vi "Set Message Methods icon without Maker.vi"() -> ()   [LabVIEW 2020]
uses:
  <vilib>/picture/picture.llb/imagedata.ctl
  <vilib>/Utility/traverseref.llb/TRef TravTarget.ctl
  <vilib>/Utility/traverseref.llb/VI Scripting - Traverse.lvlib
panel:
  in  "My Computer?":bool
  in  "Project Path":path
  out "Icon List":picture[](array[picture])
  out "Error List":string[](array[string])
  in  "Folder Path":path
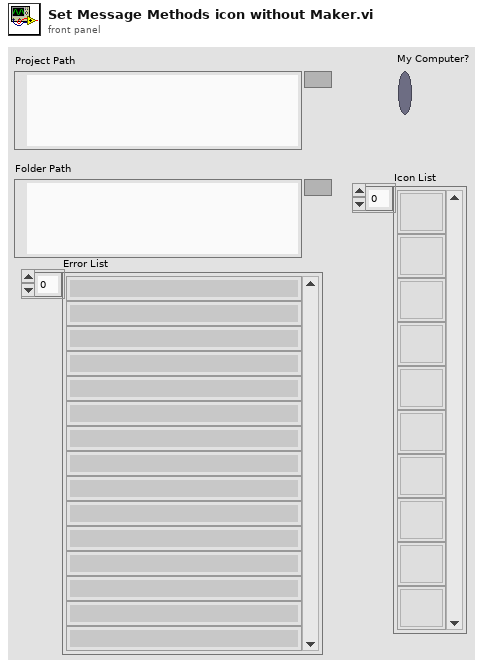
[diagram p1: front panel]
types:
  T1 = enum16{"Set Library Icon", "Get Do Core VI Icon", "Set Private Data Icon", "Set Send VI IIcon"}
  T2 = typedef "imagedata.ctl" = cluster{"image type":i32, "image depth":i32, "image":u8[], "mask":u8[], "colors":u32[], "Rectangle":cluster{"left":i16, "top":i16, "right":i16, "bottom":i16}}
  T3 = typedef "TRef TravTarget.ctl" = enum16{"FP", "BD", "Other"}
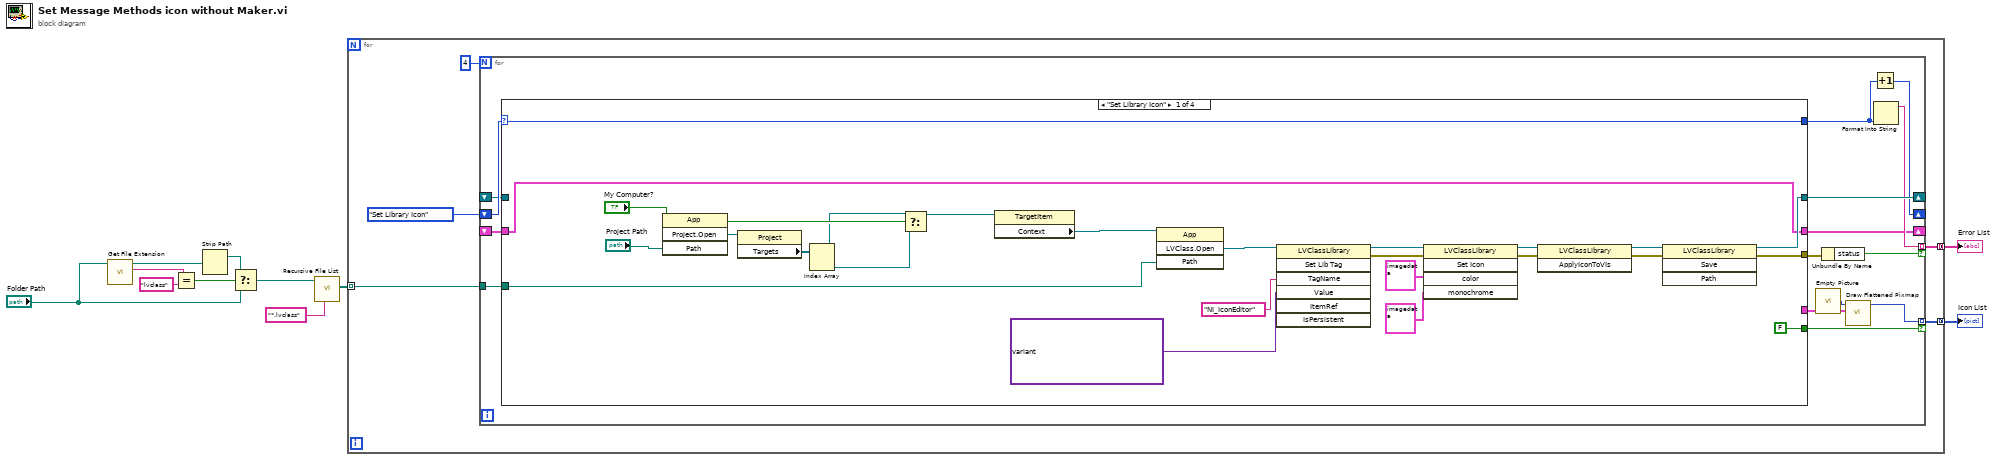
[diagram p0: block diagram]
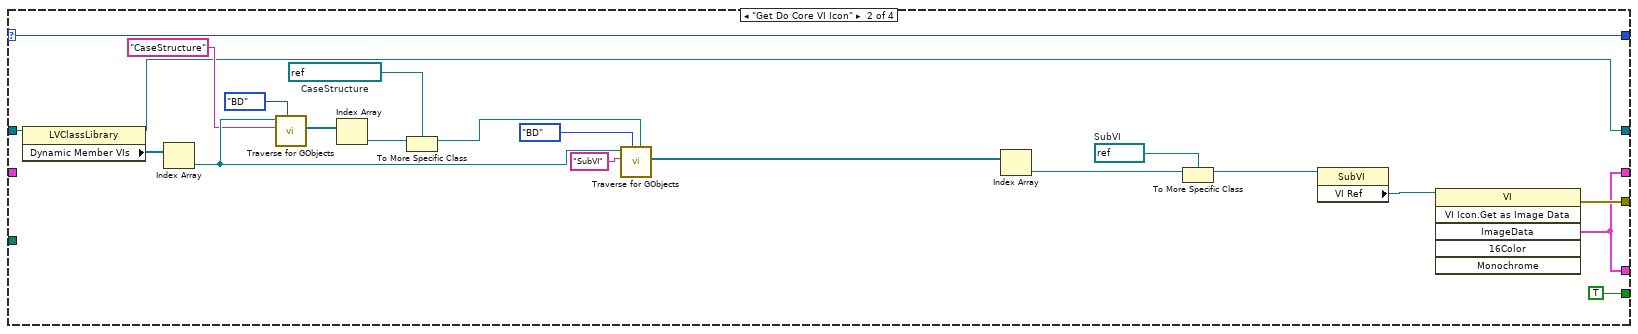
[diagram p2: hidden frame]
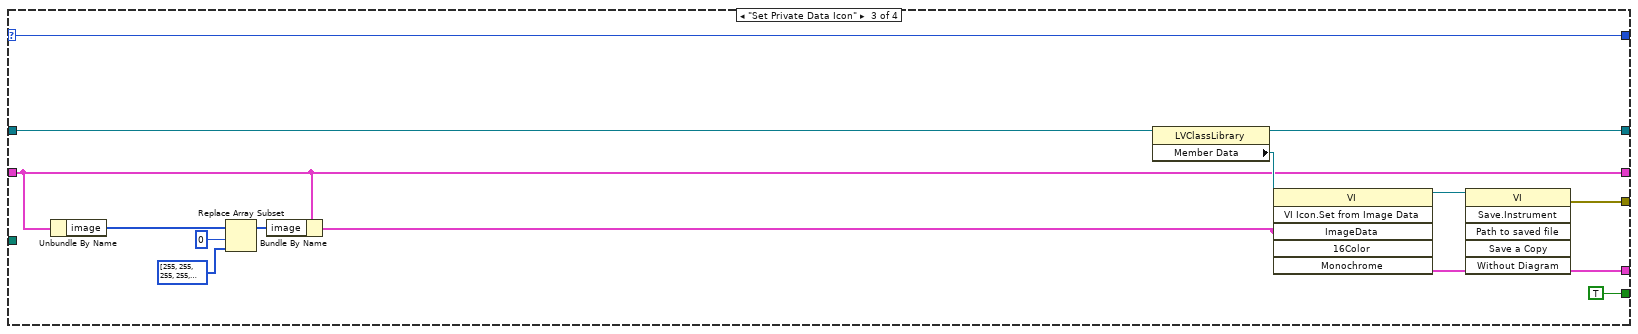
[diagram p3: hidden frame]
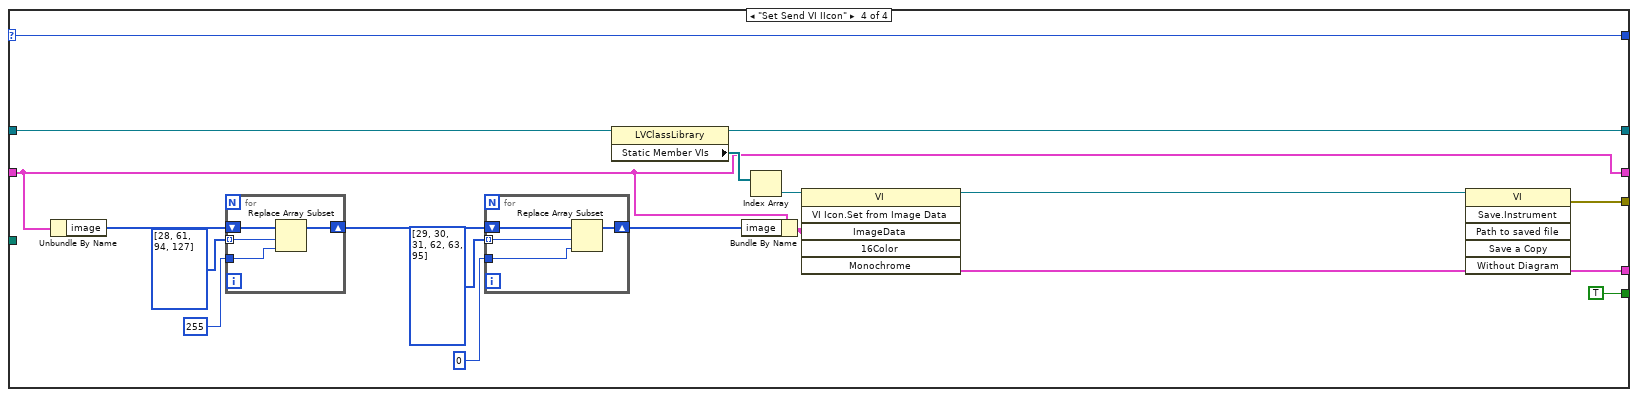
[diagram p4: hidden frame]
diagram:
  n1 = call <vilib>:"Get File Extension.vi"("file"="Folder Path") -> ("lowercase file extension"=w7:string, "dup file"=w3:path)  [unwired: 6 in, 3 out]
  n2 = Equal?(x=w7, y="lvclass") -> (x = y?=w5:bool)
  n3 = Strip Path(path=w3) -> (stripped path=w2:path)  [unwired: 1 out]
  n4 = Select(t=w2, s=w5, f="Folder Path") -> (s? t:f=w1:path)
  n5 = call <vilib>:"Recursive File List.vi"("pattern"="*.lvclass", "Folder Path"=w1) -> ("All Files in Dir"=w8:path[])  [unwired: 5 in, 4 out]
  n6 = for {
    tunnel: [w14] -> w10 mode=concatenating
    tunnel: [w13] -> w9 mode=concatenating
    tunnel: w8 -> [w12] mode=indexing
    n7 = for {
      N: 4 -> [_]
      tunnel: w12 -> [w30]
      shift-right: [w25] -> _
      shift-left: T1."Set Library Icon" -> [w31]
      shift-right: [w29] -> _
      shift-left: _ -> [w28]
      tunnel: [w27] -> w14 mode=indexing if=w20
      tunnel: [w18] -> w13 mode=indexing if=w24
      shift-right: [w23] -> _
      shift-left: _ -> [w22]
      n8 = case shown="\"Set Library Icon\"" w31 {
        selector: w31 -> [w44 w60 w78 w93]
        tunnel: w30 -> [w45 _ _ _]
        tunnel: [w44 w60 w78 w93] -> w26
        tunnel: [w43 w61 w83 w95] -> w29
        tunnel: w28 -> [_ w62 w84 w96]
        tunnel: [FALSE TRUE TRUE TRUE] -> w24
        tunnel: [w41 w57 w82 w97] -> w23
        tunnel: w22 -> [w41 _ w82 w97]
        tunnel: [w40 w58 w81 w94] -> w21
        tunnel: [_ w57 w80 w91] -> w19
        frame "Set Library Icon" {
          n9 = invoke class="App" method="Project.Open"("Path"="Project Path") -> ("Project:Open"=w38:refnum<vi>)  [unwired: 3 in, 3 out]
          n10 = property class="Project"(reference=w38) -> ("Targets"=w37:refnum<vi>[])  [unwired: 1 in, 2 out]
          n11 = Index Array(array=w37) -> (element #1=w34:refnum<vi>, element #2=w33:refnum<vi>)  [unwired: 2 in]
          n12 = Select(t=w34, s="My Computer?", f=w33) -> (s? t:f=w32:refnum<vi>)
          n13 = property class="TargetItem"(reference=w32) -> ("Context"=w39:refnum<vi>)  [unwired: 1 in, 2 out]
          n14 = invoke class="App" method="LVClass.Open"(reference=w39, "Path"=w45) -> ("LVClass.Open"=w49:refnum<vi>)  [unwired: 2 in, 3 out]
          n15 = invoke class="LVClassLibrary" method="Set Lib Tag"(reference=w49, "TagName"="NI_IconEditor" ("Tag Name"), "Value"=variant(string "49 52 48 48 56 48 51 54 13 0 0 0 0 1 23 21 76 111 97 100 32 38 32 85 110 108 111 97 100 46 108 118 99 108 97 115 115 0 0 1 0 0 0 0 0 9 0 0 5 59 1 100 1 100 80 84 72 48 0 0 0 37 0 1 0 3 5 67 108 97 115 115 11 65 99 116 111 114 32 70 114 97 109 101 14 65 70 32 77 101 115 115 97 103 101 46 112 110 103 0 0 4 206 0 40 0 0 4 200 0 0 4 128 0 0 0 0 0 12 0 32 0 24 0 0 0 0 0 255 255 255 0 0 0 0 0 0 0 0 0 0 0 0 0 0 0 0 0 0 0 0 0 0 0 0 0 0 0 0 0 0 0 0 0 0 0 0 0 0 0 0 0 0 0 0 0 0 0 0 0 0 0 0 0 0 0 0 0 0 0 0 0 0 0 0 0 0 0 0 0 0 0 0 0 0 0 0 0 0 0 0 0 0 0 0 0 0 0 0 0 0 0 0 0 0 0 0 0 0 0 0 0 153 204 255 153 204 255 153 204 255 153 204 255 153 204 255 153 204 255 153 204 255 153 204 255 153 204 255 153 204 255 153 204 255 153 204 255 153 204 255 153 204 255 153 204 255 153 204 255 153 204 255 153 204 255 153 204 255 153 204 255 153 204 255 153 204 255 153 204 255 153 204 255 153 204 255 153 204 255 153 204 255 153 204 255 153 204 255 153 204 255 0 0 0 0 0 0 153 204 255 153 204 255 153 204 255 153 204 255 153 204 255 153 204 255 153 204 255 153 204 255 153 204 255 0 0 0 0 0 0 0 0 0 0 0 0 0 0 0 0 0 0 0 0 0 0 0 0 0 0 0 0 0 0 0 0 0 0 0 0 153 204 255 153 204 255 153 204 255 153 204 255 153 204 255 153 204 255 153 204 255 153 204 255 153 204 255 0 0 0 0 0 0 153 204 255 153 204 255 153 204 255 153 204 255 153 204 255 153 204 255 153 204 255 153 204 255 153 204 255 0 0 0 153 204 255 0 0 0 0 0 0 0 0 0 0 0 0 0 0 0 0 0 0 0 0 0 0 0 0 153 204 255 0 0 0 153 204 255 153 204 255 153 204 255 153 204 255 153 204 255 153 204 255 153 204 255 153 204 255 153 204 255 0 0 0 0 0 0 153 204 255 153 204 255 153 204 255 153 204 255 153 204 255 153 204 255 153 204 255 153 204 255 153 204 255 0 0 0 0 0 0 153 204 255 0 0 0 0 0 0 0 0 0 0 0 0 0 0 0 0 0 0 153 204 255 0 0 0 0 0 0 153 204 255 153 204 255 153 204 255 153 204 255 153 204 255 153 204 255 153 204 255 153 204 255 153 204 255 0 0 0 0 0 0 153 204 255 153 204 255 153 204 255 153 204 255 153 204 255 153 204 255 153 204 255 153 204 255 153 204 255 0 0 0 0 0 0 0 0 0 153 204 255 0 0 0 0 0 0 0 0 0 0 0 0 153 204 255 0 0 0 0 0 0 0 0 0 153 204 255 153 204 255 153 204 255 153 204 255 153 204 255 153 204 255 153 204 255 153 204 255 153 204 255 0 0 0 0 0 0 153 204 255 153 204 255 153 204 255 153 204 255 153 204 255 153 204 255 153 204 255 153 204 255 153 204 255 0 0 0 0 0 0 153 204 255 0 0 0 153 204 255 0 0 0 0 0 0 153 204 255 0 0 0 153 204 255 0 0 0 0 0 0 153 204 255 153 204 255 153 204 255 153 204 255 153 204 255 153 204 255 153 204 255 153 204 255 153 204 255 0 0 0 0 0 0 153 204 255 153 204 255 153 204 255 153 204 255 153 204 255 153 204 255 153 204 255 153 204 255 153 204 255 0 0 0 153 204 255 0 0 0 0 0 0 0 0 0 153 204 255 153 204 255 0 0 0 0 0 0 0 0 0 153 204 255 0 0 0 153 204 255 153 204 255 153 204 255 153 204 255 153 204 255 153 204 255 153 204 255 153 204 255 153 204 255 0 0 0 0 0 0 153 204 255 153 204 255 153 204 255 153 204 255 153 204 255 153 204 255 153 204 255 153 204 255 153 204 255 0 0 0 0 0 0 0 0 0 0 0 0 0 0 0 0 0 0 0 0 0 0 0 0 0 0 0 0 0 0 0 0 0 0 0 0 153 204 255 153 204 255 153 204 255 153 204 255 153 204 255 153 204 255 153 204 255 153 204 255 153 204 255 0 0 0 0 0 0 153 204 255 153 204 255 153 204 255 153 204 255 153 204 255 153 204 255 153 204 255 153 204 255 153 204 255 0 0 0 0 0 0 0 0 0 0 0 0 0 0 0 0 0 0 0 0 0 0 0 0 0 0 0 0 0 0 0 0 0 0 0 0 153 204 255 153 204 255 153 204 255 153 204 255 153 204 255 153 204 255 153 204 255 153 204 255 153 204 255 0 0 0 0 0 0 153 204 255 153 204 255 153 204 255 153 204 255 153 204 255 153 204 255 153 204 255 153 204 255 153 204 255 153 204 255 153 204 255 153 204 255 153 204 255 153 204 255 153 204 255 153 204 255 153 204 255 153 204 255 153 204 255 153 204 255 153 204 255 153 204 255 153 204 255 153 204 255 153 204 255 153 204 255 153 204 255 153 204 255 153 204 255 153 204 255 0 0 0 0 0 0 0 0 0 0 0 0 0 0 0 0 0 0 0 0 0 0 0 0 0 0 0 0 0 0 0 0 0 0 0 0 0 0 0 0 0 0 0 0 0 0 0 0 0 0 0 0 0 0 0 0 0 0 0 0 0 0 0 0 0 0 0 0 0 0 0 0 0 0 0 0 0 0 0 0 0 0 0 0 0 0 0 0 0 0 0 0 0 0 0 0 0 0 0 255 255 255 255 255 255 255 255 255 255 255 255 255 255 255 255 255 255 255 255 255 255 255 255 255 255 255 255 255 255 255 255 255 255 255 255 255 255 255 255 255 255 255 255 255 255 255 255 0 0 0 0 0 0 0 0 0 0 0 0 0 0 0 0 0 0 0 0 0 0 0 0 0 0 0 0 0 0 0 0 0 0 0 0 0 0 0 11 83 109 97 108 108 32 70 111 110 116 115 0 1 10 1 0\n\n")) -> (reference out=w48:refnum<vi>, error out=w54:errorcluster)  [unwired: 4 in, 5 out]
          n16 = invoke class="LVClassLibrary" method="Set Icon"(reference=w48, error in=w54, "color"=T2 {"image type"=0, "image depth"=8, "image"=[255, 255, 255, 255, 255, 255, 255, 255, 255, 255, 255, 255, 255, 255, 255, 255, 255, 255, 255, 255, 255, 255, 255, 255, 255, 255, 255, 255, 255, 255, 255, 255, 255, 78, 78, 78, 78, 78, 78, 78, 78, 78, 78, 78, 78, 78, 78, 78, 78, 78, 78, 78, 78, 78, 78, 78, 78, 78, 78, 78, 78, 78, 78, 255, 255, 78, 78, 78, 78, 78, 78, 78, 78, 78, 255, 255, 255, 255, 255, 255, 255, 255, 255, 255, 255, 255, 78, 78, 78, 78, 78, 78, 78, 78, 78, 255, 255, 78, 78, 78, 78, 78, 78, 78, 78, 78, 255, 78, 255, 255, 255, 255, 255, 255, 255, 255, 78, 255, 78, 78, 78, 78, 78, 78, 78, 78, 78, 255, 255, 78, 78, 78, 78, 78, 78, 78, 78, 78, 255, 255, 78, 255, 255, 255, 255, 255, 255, 78, 255, 255, 78, 78, 78, 78, 78, 78, 78, 78, 78, 255, 255, 78, 78, 78, 78, 78, 78, 78, 78, 78, 255, 255, 255, 78, 255, 255, 255, 255, 78, 255, 255, 255, 78, 78, 78, 78, 78, 78, 78, 78, 78, 255, 255, 78, 78, 78, 78, 78, 78, 78, 78, 78, 255, 255, 78, 255, 78, 255, 255, 78, 255, 78, 255, 255, 78, 78, 78, 78, 78, 78, 78, 78, 78, 255, 255, 78, 78, 78, 78, 78, 78, 78, 78, 78, 255, 78, 255, 255, 255, 78, 78, 255, 255, 255, 78, 255, 78, 78, 78, 78, 78, 78, 78, 78, 78, 255, 255, 78, 78, 78, 78, 78, 78, 78, 78, 78, 255, 255, 255, 255, 255, 255, 255, 255, 255, 255, 255, 255, 78, 78, 78, 78, 78, 78, 78, 78, 78, 255, 255, 78, 78, 78, 78, 78, 78, 78, 78, 78, 255, 255, 255, 255, 255, 255, 255, 255, 255, 255, 255, 255, 78, 78, 78, 78, 78, 78, 78, 78, 78, 255, 255, 78, 78, 78, 78, 78, 78, 78, 78, 78, 78, 78, 78, 78, 78, 78, 78, 78, 78, 78, 78, 78, 78, 78, 78, 78, 78, 78, 78, 78, 78, 255, 255, 255, 255, 255, 255, 255, 255, 255, 255, 255, 255, 255, 255, 255, 255, 255, 255, 255, 255, 255, 255, 255, 255, 255, 255, 255, 255, 255, 255, 255, 255, 255, 0, 0, 0, 0, 0, 0, 0, 0, 0, 0, 0, 0, 0, 0, 0, 0, 0, 0, 0, 0, 0, 0, 0, 0, 0, 0, 0, 0, 0, 0, 0, 0, 0, 0, 0, 0, 0, 0, 0, 0, 0, 0, 0, 0, 0, 0, 0, 0, 0, 0, 0, 0, 0, 0, 0, 0, 0, 0, 0, 0, 0, 0, 0, 0, 0, 0, 0, 0, 0, 0, 0, 0, 0, 0, 0, 0, 0, 0, 0, 0, 0, 0, 0, 0, 0, 0, 0, 0, 0, 0, 0, 0, 0, 0, 0, 0, 0, 0, 0, 0, 0, 0, 0, 0, 0, 0, 0, 0, 0, 0, 0, 0, 0, 0, 0, 0, 0, 0, 0, 0, 0, 0, 0, 0, 0, 0, 0, 0, 0, 0, 0, 0, 0, 0, 0, 0, 0, 0, 0, 0, 0, 0, 0, 0, 0, 0, 0, 0, 0, 0, 0, 0, 0, 0, 0, 0, 0, 0, 0, 0, 0, 0, 0, 0, 0, 0, 0, 0, 0, 0, 0, 0, 0, 0, 0, 0, 0, 0, 0, 0, 0, 0, 0, 0, 0, 0, 0, 0, 0, 0, 0, 0, 0, 0, 0, 0, 0, 0, 0, 0, 0, 0, 0, 0, 0, 0, 0, 0, 0, 0, 0, 0, 0, 0, 0, 0, 0, 0, 0, 0, 0, 0, 0, 0, 0, 0, 0, 0, 0, 0, 0, 0, 0, 0, 0, 0, 0, 0, 0, 0, 0, 0, 0, 0, 0, 0, 0, 0, 0, 0, 0, 0, 0, 0, 0, 0, 0, 0, 0, 0, 0, 0, 0, 0, 0, 0, 0, 0, 0, 0, 0, 0, 0, 0, 0, 0, 0, 0, 0, 0, 0, 0, 0, 0, 0, 0, 0, 0, 0, 0, 0, 0, 0, 0, 0, 0, 0, 0, 0, 0, 0, 0, 0, 0, 0, 0, 0, 0, 0, 0, 0, 0, 0, 0, 0, 0, 0, 0, 0, 0, 0, 0, 0, 0, 0, 0, 0, 0, 0, 0, 0, 0, 0, 0, 0, 0, 0, 0, 0, 0, 0, 0, 0, 0, 0, 0, 0, 0, 0, 0, 0, 0, 0, 0, 0, 0, 0, 0, 0, 0, 0, 0, 0, 0, 0, 0, 0, 0, 0, 0, 0, 0, 0, 0, 0, 0, 0, 0, 0, 0, 0, 0, 0, 0, 0, 0, 0, 0, 0, 0, 0, 0, 0, 0, 0, 0, 0, 0, 0, 0, 0, 0, 0, 0, 0, 0, 0, 0, 0, 0, 0, 0, 0, 0, 0, 0, 0, 0, 0, 0, 0, 0, 0, 0, 0, 0, 0, 0, 0, 0, 0, 0, 0, 0, 0, 0, 0, 0, 0, 0, 0, 0, 0, 0, 0, 0, 0, 0, 0, 0, 0, 0, 0, 0, 0, 0, 0, 0, 0, 0, 0, 0, 0, 0, 0, 0, 0, 0, 0, 0, 0, 0, 0, 0, 0, 0, 0, 0, 0, 0, 0, 0, 0, 0, 0, 0, 0, 0, 0, 0, 0, 0, 0, 0, 0, 0, 0, 0, 0, 0, 0, 0, 0, 0, 0, 0, 0, 0, 0, 0, 0, 0, 0, 0, 0, 0, 0, 0, 0, 0, 0, 0, 0, 0, 0, 0, 0, 0, 0, 0, 0, 0, 0, 0, 0, 0, 0, 0, 0, 0, 0, 0, 0, 0, 0, 0, 0, 0, 0, 0, 0, 0, 0, 0, 0, 0, 0, 0, 0, 0, 0, 0, 0, 0, 0, 0, 0, 0, 0, 0, 0, 0, 0, 0, 0, 0, 0, 0, 0, 0, 0, 0, 0, 0, 0, 0, 0, 0, 0, 0, 0, 0, 0, 0, 0, 0, 0, 0, 0, 0, 0, 0, 0, 0, 0, 0, 0, 0, 0, 0, 0, 0, 0, 0, 0, 0, 0, 0, 0, 0, 0, 0, 0, 0, 0, 0, 0, 0, 0, 0, 0, 0, 0, 0, 0, 0, 0, 0, 0, 0], "mask"=[255, 255, 255, 255, 255, 255, 255, 255, 255, 255, 255, 255, 255, 255, 255, 255, 255, 255, 255, 255, 255, 255, 255, 255, 255, 255, 255, 255, 255, 255, 255, 255, 255, 255, 255, 255, 255, 255, 255, 255, 255, 255, 255, 255, 255, 255, 255, 255, 0, 0, 0, 0, 0, 0, 0, 0, 0, 0, 0, 0, 0, 0, 0, 0, 0, 0, 0, 0, 0, 0, 0, 0, 0, 0, 0, 0, 0, 0, 0, 0, 0, 0, 0, 0, 0, 0, 0, 0, 0, 0, 0, 0, 0, 0, 0, 0, 0, 0, 0, 0, 0, 0, 0, 0, 0, 0, 0, 0, 0, 0, 0, 0, 0, 0, 0, 0, 0, 0, 0, 0, 0, 0, 0, 0, 0, 0, 0, 0], "colors"=[16777215, 16777164, 16777113, 16777062, 16777011, 16776960, 16764159, 16764108, 16764057, 16764006, 16763955, 16763904, 16751103, 16751052, 16751001, 16750950, 16750899, 16750848, 16738047, 16737996, 16737945, 16737894, 16737843, 16737792, 16724991, 16724940, 16724889, 16724838, 16724787, 16724736, 16711935, 16711884, 16711833, 16711782, 16711731, 16711680, 13434879, 13434828, 13434777, 13434726, 13434675, 13434624, 13421823, 13421772, 13421721, 13421670, 13421619, 13421568, 13408767, 13408716, 13408665, 13408614, 13408563, 13408512, 13395711, 13395660, 13395609, 13395558, 13395507, 13395456, 13382655, 13382604, 13382553, 13382502, 13382451, 13382400, 13369599, 13369548, 13369497, 13369446, 13369395, 13369344, 10092543, 10092492, 10092441, 10092390, 10092339, 10092288, 10079487, 10079436, 10079385, 10079334, 10079283, 10079232, 10066431, 10066380, 10066329, 10066278, 10066227, 10066176, 10053375, 10053324, 10053273, 10053222, 10053171, 10053120, 10040319, 10040268, 10040217, 10040166, 10040115, 10040064, 10027263, 10027212, 10027161, 10027110, 10027059, 10027008, 6750207, 6750156, 6750105, 6750054, 6750003, 6749952, 6737151, 6737100, 6737049, 6736998, 6736947, 6736896, 6724095, 6724044, 6723993, 6723942, 6723891, 6723840, 6711039, 6710988, 6710937, 6710886, 6710835, 6710784, 6697983, 6697932, 6697881, 6697830, 6697779, 6697728, 6684927, 6684876, 6684825, 6684774, 6684723, 6684672, 3407871, 3407820, 3407769, 3407718, 3407667, 3407616, 3394815, 3394764, 3394713, 3394662, 3394611, 3394560, 3381759, 3381708, 3381657, 3381606, 3381555, 3381504, 3368703, 3368652, 3368601, 3368550, 3368499, 3368448, 3355647, 3355596, 3355545, 3355494, 3355443, 3355392, 3342591, 3342540, 3342489, 3342438, 3342387, 3342336, 65535, 65484, 65433, 65382, 65331, 65280, 52479, 52428, 52377, 52326, 52275, 52224, 39423, 39372, 39321, 39270, 39219, 39168, 26367, 26316, 26265, 26214, 26163, 26112, 13311, 13260, 13209, 13158, 13107, 13056, 255, 204, 153, 102, 51, 15597568, 14483456, 12255232, 11141120, 8912896, 7798784, 5570560, 4456448, 2228224, 1114112, 60928, 56576, 47872, 43520, 34816, 30464, 21760, 17408, 8704, 4352, 238, 221, 187, 170, 136, 119, 85, 68, 34, 17, 15658734, 14540253, 12303291, 11184810, 8947848, 7829367, 5592405, 4473924, 2236962, 1118481, 0], "Rectangle"={"left"=0, "top"=0, "right"=32, "bottom"=32}}, "monochrome"=T2 {"image type"=0, "image depth"=1, "image"=[255, 255, 255, 255, 128, 0, 0, 1, 128, 63, 252, 1, 128, 47, 244, 1, 128, 55, 236, 1, 128, 59, 220, 1, 128, 53, 172, 1, 128, 46, 116, 1, 128, 63, 252, 1, 128, 63, 252, 1, 128, 0, 0, 1, 255, 255, 255, 255, 0, 0, 0, 0, 0, 0, 0, 0, 0, 0, 0, 0, 0, 0, 0, 0, 0, 0, 0, 0, 0, 0, 0, 0, 0, 0, 0, 0, 0, 0, 0, 0, 0, 0, 0, 0, 0, 0, 0, 0, 0, 0, 0, 0, 0, 0, 0, 0, 0, 0, 0, 0, 0, 0, 0, 0, 0, 0, 0, 0, 0, 0, 0, 0, 0, 0, 0, 0, 0, 0, 0, 0, 0, 0, 0, 0, 0, 0, 0, 0], "mask"=[255, 255, 255, 255, 255, 255, 255, 255, 255, 255, 255, 255, 255, 255, 255, 255, 255, 255, 255, 255, 255, 255, 255, 255, 255, 255, 255, 255, 255, 255, 255, 255, 255, 255, 255, 255, 255, 255, 255, 255, 255, 255, 255, 255, 255, 255, 255, 255, 0, 0, 0, 0, 0, 0, 0, 0, 0, 0, 0, 0, 0, 0, 0, 0, 0, 0, 0, 0, 0, 0, 0, 0, 0, 0, 0, 0, 0, 0, 0, 0, 0, 0, 0, 0, 0, 0, 0, 0, 0, 0, 0, 0, 0, 0, 0, 0, 0, 0, 0, 0, 0, 0, 0, 0, 0, 0, 0, 0, 0, 0, 0, 0, 0, 0, 0, 0, 0, 0, 0, 0, 0, 0, 0, 0, 0, 0, 0, 0], "colors"=[16777215, 0], "Rectangle"={"left"=0, "top"=0, "right"=32, "bottom"=32}}) -> (reference out=w47:refnum<vi>, error out=w55:errorcluster)  [unwired: 1 in, 3 out]
          n17 = invoke class="LVClassLibrary" method="ApplyIconToVIs"(reference=w47, error in=w55) -> (reference out=w46:refnum<vi>, error out=w56:errorcluster)  [unwired: 1 in, 1 out]
          n18 = invoke class="LVClassLibrary" method="Save"(reference=w46, error in=w56) -> (reference out=w43:refnum<vi>, error out=w40:errorcluster)  [unwired: 2 in, 2 out]
        }
        frame "Get Do Core VI Icon" {
          w69 = refnum<vi> refnum  # SubVI
          w67 = refnum<vi> refnum  # CaseStructure
          n19 = property class="LVClassLibrary"(reference=w62) -> (reference out=w61:refnum<vi>, "Dynamic Member VIs"=w63:refnum<vi>[])  [unwired: 1 in, 1 out]
          n20 = Index Array(array=w63) -> (element=w74:refnum<vi>)  [unwired: 1 in]
          n21 = call <vilib>:"Traverse for GObjects.vi"("Traverse Target"=TRef_TravTarget."BD", "Class Name"="CaseStructure", "VI Refnum"=w74) -> ("References"=w71:refnum<vi>[])  [unwired: 5 in, 3 out]
          n22 = Index Array(array=w71) -> (element=w66:refnum<vi>)  [unwired: 1 in]
          n23 = To More Specific Class(target class=w67, reference=w66) -> (specific class reference=w75:refnum<vi>)  [unwired: 1 in, 1 out]
          n24 = call <vilib>:"Traverse for GObjects.vi"("Other Refnum"=w75, "Traverse Target"=TRef_TravTarget."BD", "Class Name"="SubVI", "VI Refnum"=w74) -> ("References"=w73:refnum<vi>[])  [unwired: 4 in, 3 out]
          n25 = Index Array(array=w73) -> (element=w72:refnum<vi>)  [unwired: 1 in]
          n26 = To More Specific Class(target class=w69, reference=w72) -> (specific class reference=w68:refnum<vi>)  [unwired: 1 in, 1 out]
          n27 = property class="SubVI"(reference=w68) -> ("VI Ref"=w70:refnum<vi>)  [unwired: 1 in, 2 out]
          n28 = invoke class="VI" method="VI Icon.Get as Image Data"(reference=w70) -> (error out=w58:errorcluster, "ImageData"=w57:T2)  [unwired: 5 in, 4 out]
        }
        frame "Set Private Data Icon" {
          n29 = Unbundle By Name(w82) -> ("image"=w90:u8[])
          n30 = Replace Array Subset(array=w90, new element=u8[] [255, 255, 255, 255, 255, 255, 255, 255, 255, 255, 255, 255, 255, 255, 255, 255, 255, 255, 255, 255, 255, 255, 255, 255, 255, 255, 255, 255, 255, 255, 255, 255, 255, 0, 0, 0, 0, 0, 0, 0, 0, 0, 0, 0, 0, 0, 0, 0, 0, 0, 0, 0, 0, 0, 0, 0, 0, 0, 0, 0, 0, 0, 0, 255, 255, 0, 0, 0, 0, 0, 0, 0, 0, 0, 0, 0, 0, 0, 0, 0, 0, 0, 0, 0, 0, 0, 0, 0, 0, 0, 0, 0, 0, 0, 0, 255, 255, 0, 0, 0, 0, 0, 0, 0, 0, 0, 0, 0, 0, 0, 0, 0, 0, 0, 0, 0, 0, 0, 0, 0, 0, 0, 0, 0, 0, 0, 0, 255, 255, 0, 0, 0, 0, 0, 0, 0, 0, 0, 0, 0, 0, 0, 0, 0, 0, 0, 0, 0, 0, 0, 0, 0, 0, 0, 0, 0, 0, 0, 0, 255, 255, 0, 0, 0, 0, 0, 0, 0, 0, 0, 0, 0, 0, 0, 0, 0, 0, 0, 0, 0, 0, 0, 0, 0, 0, 0, 0, 0, 0, 0, 0, 255, 255, 0, 0, 0, 0, 0, 0, 0, 0, 0, 0, 0, 0, 0, 0, 0, 0, 0, 0, 0, 0, 0, 0, 0, 0, 0, 0, 0, 0, 0, 0, 255, 255, 0, 0, 0, 0, 0, 0, 0, 0, 0, 0, 0, 0, 0, 0, 0, 0, 0, 0, 0, 0, 0, 0, 0, 0, 0, 0, 0, 0, 0, 0, 255, 255, 0, 0, 0, 0, 0, 0, 0, 0, 0, 0, 0, 0, 0, 0, 0, 0, 0, 0, 0, 0, 0, 0, 0, 0, 0, 0, 0, 0, 0, 0, 255, 255, 0, 0, 0, 0, 0, 0, 0, 0, 0, 0, 0, 0, 0, 0, 0, 0, 0, 0, 0, 0, 0, 0, 0, 0, 0, 0, 0, 0, 0, 0, 255, 255, 0, 0, 0, 0, 0, 0, 0, 0, 0, 0, 0, 0, 0, 0, 0, 0, 0, 0, 0, 0, 0, 0, 0, 0, 0, 0, 0, 0, 0, 0, 255, 255, 0, 0, 0, 0, 0, 0, 0, 0, 0, 0, 0, 0, 0, 0, 0, 0, 0, 0, 0, 0, 0, 0, 0, 0, 0, 0, 0, 0, 0, 0, 255] ("subarray"), index=0) -> (w87:u8[])
          n31 = Bundle By Name(cluster=w82, "image"=w87) -> (w80:T2)
          n32 = property class="LVClassLibrary"(reference=w84) -> (reference out=w83:refnum<vi>, "Member Data"=w86:refnum<vi>)  [unwired: 1 in, 1 out]
          n33 = invoke class="VI" method="VI Icon.Set from Image Data"(reference=w86, "ImageData"=w80) -> (reference out=w85:refnum<vi>)  [unwired: 4 in, 5 out]
          n34 = invoke class="VI" method="Save.Instrument"(reference=w85) -> (error out=w81:errorcluster)  [unwired: 5 in, 5 out]
        }
        frame "Set Send VI IIcon" {
          n35 = Unbundle By Name(w97) -> ("image"=w98:u8[])
          n36 = for {
            tunnel: u8 255 ("new element/subarray") -> [w114]
            shift-right: [w113] -> w105
            shift-left: w98 -> [w115]
            tunnel: i32[] [28, 61, 94, 127] -> [w112] mode=indexing
            n37 = Replace Array Subset(array=w115, new element=w114, index=w112) -> (w113:u8[])
          }
          n38 = for {
            tunnel: u8 0 ("new element/subarray") -> [w110]
            shift-right: [w109] -> w102
            shift-left: w105 -> [w111]
            tunnel: i32[] [29, 30, 31, 62, 63, 95] -> [w108] mode=indexing
            n39 = Replace Array Subset(array=w111, new element=w110, index=w108) -> (w109:u8[])
          }
          n40 = property class="LVClassLibrary"(reference=w96) -> (reference out=w95:refnum<vi>, "Static Member VIs"=w101:refnum<vi>[])  [unwired: 1 in, 1 out]
          n41 = Bundle By Name(cluster=w97, "image"=w102) -> (w91:T2)
          n42 = Index Array(array=w101) -> (element=w100:refnum<vi>)  [unwired: 1 in]
          n43 = invoke class="VI" method="VI Icon.Set from Image Data"(reference=w100, "ImageData"=w91) -> (reference out=w99:refnum<vi>)  [unwired: 4 in, 5 out]
          n44 = invoke class="VI" method="Save.Instrument"(reference=w99) -> (error out=w94:errorcluster)  [unwired: 5 in, 5 out]
        }
      }
      n45 = call "Empty Picture"() -> ("empty picture"=w17:picture)
      n46 = Unbundle By Name(w21) -> ("status"=w20:bool)
      n47 = call <vilib>:"Draw Flattened Pixmap.vi"("image data"=w19, "picture"=w17) -> ("new picture"=w18:picture)  [unwired: 7 in]
      n48 = Increment(x=w26) -> (x+1=w25:T1)
      n49 = Format Into String(w26) -> (resulting string=w27:string)  [unwired: 3 in, 1 out]
    }
  }
  "Error List" <- w10
  "Icon List" <- w9
